vi "indice de comida.vi"(11 "NewVal":T1) -> (3 "Numeric":dbl)   [LabVIEW 2015]
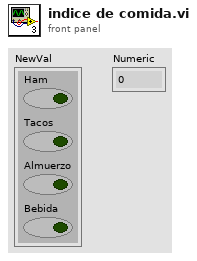
[diagram p1: front panel]
types:
  T1 = cluster{"Ham":bool, "Tacos":bool, "Almuerzo":bool, "Bebida":bool}
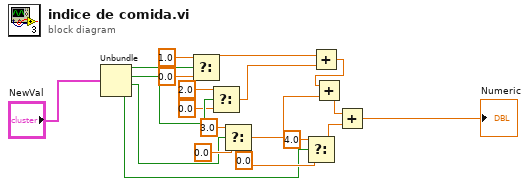
[diagram p0: block diagram]
diagram:
  n1 = Unbundle("NewVal") -> ("Ham"=w2:bool, "Tacos"=w8:bool, "Almuerzo"=w9:bool, "Bebida"=w11:bool)
  n2 = Select(t=1.0, s=w2, f=0.0) -> (s? t:f=w14:dbl)
  n3 = Select(t=2.0, s=w8, f=0.0) -> (s? t:f=w15:dbl)
  n4 = Select(t=3.0, s=w9, f=0.0) -> (s? t:f=w17:dbl)
  n5 = Select(t=4.0, s=w11, f=0.0) -> (s? t:f=w19:dbl)
  n6 = Add(x=w14, y=w15) -> (x+y=w16:dbl)
  n7 = Add(x=w16, y=w17) -> (x+y=w18:dbl)
  n8 = Add(x=w18, y=w19) -> (x+y=→"Numeric":dbl)
